vi "Stretch Pulse (Fixed).vi"(11 "Pulse":bool) -> (3 "Stretched Pulse":bool)   [LabVIEW 2012]
doc: "This VI stretches a pulse by 4 Ticks. This is useful when send triggers on PXI_Trig lines."
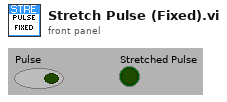
[diagram p1: front panel]
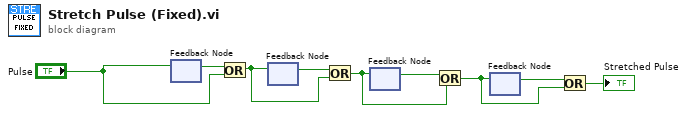
[diagram p0: block diagram]
diagram:
  n1 = feedback #1() -> (w9:bool)  [unwired: 1 in]
  n2 = feedback-in #1("Pulse") -> ()
  n3 = Or(x=w9, y="Pulse") -> (x .or. y?=w5:bool)
  n4 = feedback #2() -> (w8:bool)  [unwired: 1 in]
  n5 = feedback-in #2(w5) -> ()
  n6 = Or(x=w8, y=w5) -> (x .or. y?=w4:bool)
  n7 = feedback #3() -> (w6:bool)  [unwired: 1 in]
  n8 = feedback-in #3(w4) -> ()
  n9 = Or(x=w6, y=w4) -> (x .or. y?=w3:bool)
  n10 = feedback #4() -> (w7:bool)  [unwired: 1 in]
  n11 = feedback-in #4(w3) -> ()
  n12 = Or(x=w7, y=w3) -> (x .or. y?=→"Stretched Pulse":bool)
